vi "Example - Type Assertion.vi"() -> ()   [LabVIEW 2020]
uses:
  5ade6ed0-875b-3fb7-d487-db305fe8d93f.vi
  a13809fc-20bb-3fe1-f8e7-b7c2f04bc43f.vi
  Robot/Robot.lvclass
  EquipmentVariant/EquipmentVariant.lvclass
  home/jki/Projects/enumerated-variant-labview-idea/source/EnumeratedVariant/EnumeratedVariant.lvclass
  home/jki/Projects/enumerated-variant-labview-idea/source/EquipmentVariant/EquipmentVariant.lvclass
  EquipmentVariant/Type Enum.ctl
  Pump/Pump.lvclass
panel:
  out "Type Enum out":T1=enum."Instrument"
  in  "Type":refnum<class "Robot.lvclass">
  out "Specific Variant":refnum<class "Robot.lvclass">
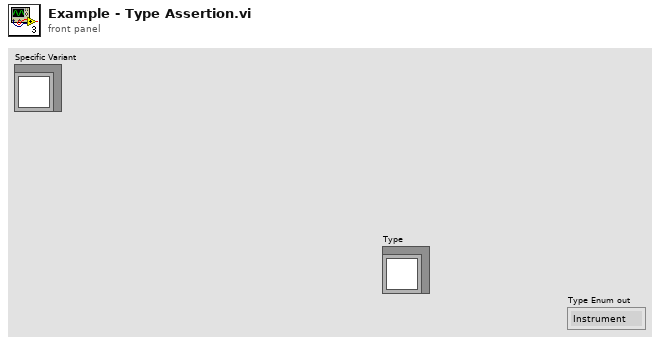
[diagram p1: front panel]
types:
  T1 = typedef "EquipmentVariant.lvclass/Type Enum.ctl" = enum16{"Robot", "Pump", "Instrument"}
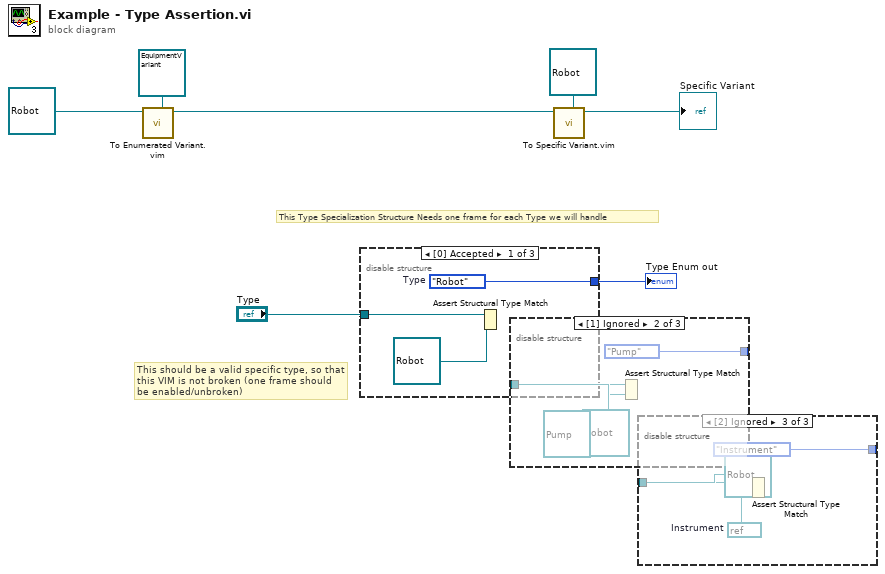
[diagram p0: block diagram]
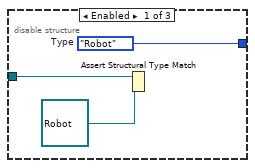
[diagram p2: hidden frame]
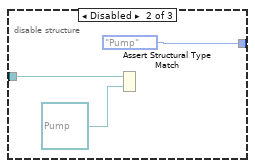
[diagram p3: hidden frame]
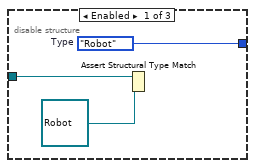
[diagram p4: hidden frame]
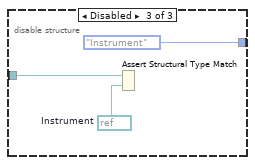
[diagram p5: hidden frame]
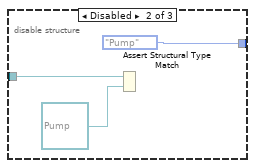
[diagram p6: hidden frame]
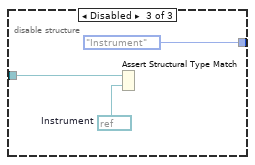
[diagram p7: hidden frame]
diagram:
  # "This should be a valid specific type, so that this VIM is not broken (one frame should be enabled/unbroken)"
  # "This Type Specialization Structure Needs one frame for each Type we will handle"
  n1 = call "To Enumerated Variant.vim"("Enumerated Type"=refnum<class "EquipmentVariant.lvclass"> refnum, "Type"=refnum<class "Robot.lvclass"> refnum) -> ("EquipmentVariant"=w6:refnum<class "EquipmentVariant.lvclass">)  [unwired: 8 in, 1 out]
  n2 = disable-structure shown="[0] Accepted" {
    disable-tunnel: "Type" -> [w12 w15 w18]
    disable-tunnel: [w11 Type_Enum."Pump" ("Type") Type_Enum."Instrument" ("Type")] -> w3
    frame Enabled {
      w11 = Type_Enum."Robot"  # Type
      n3 = Assert Structural Type Match(0:refnum<class "Robot.lvclass"> refnum ("Robot.lvclass"), 1:w12) -> ()
    }
    frame Disabled {
      n4 = Assert Structural Type Match(0:refnum<class "Pump.lvclass"> refnum ("Pump.lvclass"), 1:w15) -> ()
    }
    frame Disabled {
      w17 = refnum<visa-resource-name> refnum  # Instrument
      n5 = Assert Structural Type Match(0:w17, 1:w18) -> ()
    }
  }
  "Type Enum out" <- w3
  n6 = disable-structure shown="[1] Ignored" {
    disable-tunnel: refnum<class "Robot.lvclass"> refnum ("Type 2") -> [w21 w24 w27]
    disable-tunnel: [w20 Type_Enum."Pump" ("Type") Type_Enum."Instrument" ("Type")] -> _
    frame Enabled {
      w20 = Type_Enum."Robot"  # Type
      n7 = Assert Structural Type Match(0:refnum<class "Robot.lvclass"> refnum ("Robot.lvclass"), 1:w21) -> ()
    }
    frame Disabled {
      n8 = Assert Structural Type Match(0:refnum<class "Pump.lvclass"> refnum ("Pump.lvclass"), 1:w24) -> ()
    }
    frame Disabled {
      w26 = refnum<visa-resource-name> refnum  # Instrument
      n9 = Assert Structural Type Match(0:w26, 1:w27) -> ()
    }
  }
  n10 = call "To Specific Variant.vim"("Type"=refnum<class "Robot.lvclass"> refnum, "EquipmentVariant.lvclass"=w6) -> ("Specific Variant"=→"Specific Variant":refnum<class "Robot.lvclass">)  [unwired: 8 in, 1 out]
  n11 = disable-structure shown="[2] Ignored" {
    disable-tunnel: refnum<class "Robot.lvclass"> refnum ("Type 3") -> [w30 w33 w36]
    disable-tunnel: [w29 Type_Enum."Pump" ("Type") Type_Enum."Instrument" ("Type")] -> _
    frame Enabled {
      w29 = Type_Enum."Robot"  # Type
      n12 = Assert Structural Type Match(0:refnum<class "Robot.lvclass"> refnum ("Robot.lvclass"), 1:w30) -> ()
    }
    frame Disabled {
      n13 = Assert Structural Type Match(0:refnum<class "Pump.lvclass"> refnum ("Pump.lvclass"), 1:w33) -> ()
    }
    frame Disabled {
      w35 = refnum<visa-resource-name> refnum  # Instrument
      n14 = Assert Structural Type Match(0:w35, 1:w36) -> ()
    }
  }
